vi "Rotate.vi"(8 "error in (no error)":errorcluster, 10 "Angle (deg)":dbl, 11 "Collection in":refnum<class "Collection.lvclass">) -> (0 "error out":errorcluster, 3 "Collection out":refnum<class "Collection.lvclass">)   [LabVIEW 2021, in "Picture2D.lvlib" / "Collection.lvclass"]
uses:
  Collection.lvclass
  Collection.lvclass/Collection.ctl
  IDrawable/IDrawable.lvclass
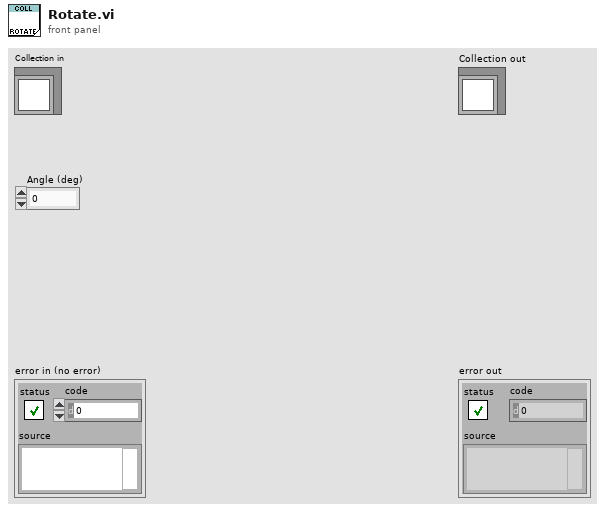
[diagram p1: front panel]
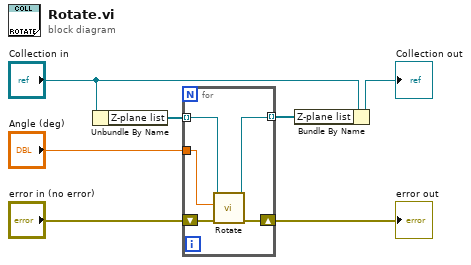
[diagram p0: block diagram]
diagram:
  n1 = Unbundle By Name("Collection in") -> ("Z-plane list"=w7:refnum<class "IDrawable.lvclass">[])
  n2 = for {
    tunnel: w7 -> [w12] mode=indexing
    tunnel: "Angle (deg)" -> [w8]
    tunnel: [w11] -> w5 mode=indexing
    shift-right: [w9] -> w1
    shift-left: "error in (no error)" -> [w10]
    n3 = call-dynamic "Rotate.vi"("error in (no error)"=w10, "Angle (deg)"=w8, "IRotatable in"=w12) -> ("error out"=w9:errorcluster, "IRotatable out"=w11:refnum<class "IDrawable.lvclass">)  [unwired: 7 in]
  }
  "error out" <- w1
  n4 = Bundle By Name(cluster="Collection in", "Z-plane list"=w5) -> (→"Collection out":refnum<class "Collection.lvclass">)
